vi "Keep String Num same length.vi"(7 "length":i32, 11 "Str Num":string) -> (3 "Str Num (same length)":string)   [LabVIEW 2021]
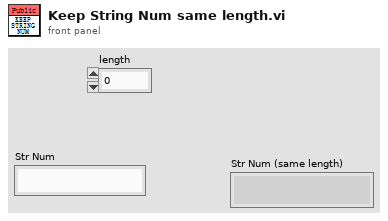
[diagram p1: front panel]
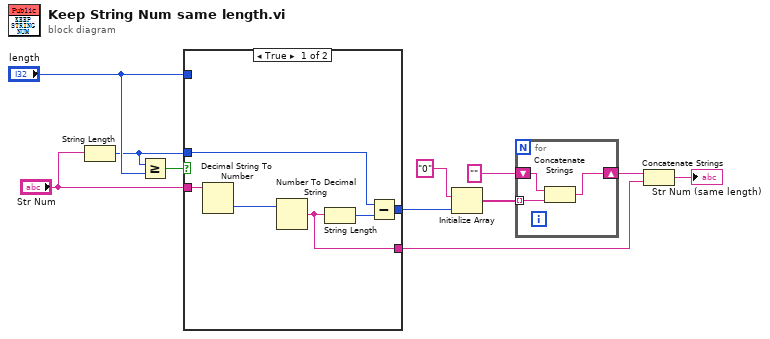
[diagram p0: block diagram]
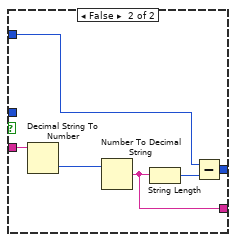
[diagram p2: hidden frame]
diagram:
  n1 = String Length(string="Str Num") -> (length=w9:i32)
  n2 = Greater Or Equal?(x=w9, y="length") -> (x >= y?=w10:bool)
  n3 = case shown="True" w10 {
    tunnel: [w17 w23] -> w2
    tunnel: [w16 w22] -> w6
    tunnel: "Str Num" -> [w15 w21]
    tunnel: w9 -> [w13 _]
    tunnel: "length" -> [_ w19]
    frame True {
      n4 = Decimal String To Number(string=w15) -> (number=w12:i32)  [unwired: 2 in, 1 out]
      n5 = Number To Decimal String(number=w12) -> (decimal integer string=w16:string)  [unwired: 1 in]
      n6 = String Length(string=w16) -> (length=w14:i32)
      n7 = Subtract(x=w13, y=w14) -> (x-y=w17:i32)
    }
    frame False {
      n8 = Decimal String To Number(string=w21) -> (number=w18:i32)  [unwired: 2 in, 1 out]
      n9 = Number To Decimal String(number=w18) -> (decimal integer string=w22:string)  [unwired: 1 in]
      n10 = String Length(string=w22) -> (length=w20:i32)
      n11 = Subtract(x=w19, y=w20) -> (x-y=w23:i32)
    }
  }
  n12 = Initialize Array("0" ("substring"), w2) -> (w3:string[])
  n13 = for {
    tunnel: w3 -> [w26] mode=indexing
    shift-right: [w24] -> w5
    shift-left: "" ("s? t:f") -> [w25]
    n14 = Concatenate Strings(w25, w26) -> (w24:string)
  }
  n15 = Concatenate Strings(w5, w6) -> (→"Str Num (same length)":string)
